vi "Frame create.vi"(7 "Command":string, 8 "error in (no error)":errorcluster, 11 "ISO 14443 B DOWN in":refnum<class "ISO 14443 B DOWN.lvclass">) -> (0 "error out":errorcluster, 3 "ISO 14443 B DOWN out":refnum<class "ISO 14443 B DOWN.lvclass">)   [LabVIEW 2019, in "ISO 14443 B DOWN.lvclass"]
uses:
  ISO 14443 B DOWN.lvclass
  TypeDef/Store.ctl
  ISO 14443 B DOWN.lvclass/ISO 14443 B DOWN.ctl
  RFID system.lvclass
panel:
  in  "APf":u8[](array[numeric])=[5] format="%x"
  in  "AFi":u8[](array[numeric])=[2] format="%x"
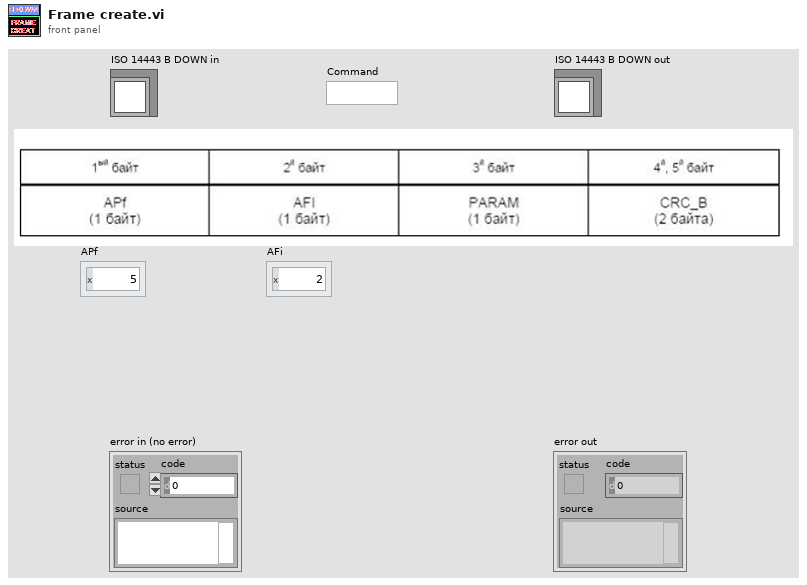
[diagram p1: front panel]
types:
  T1 = typedef "Store.ctl" = enum16{"envelope", "noise", "demSubCar", "CH_frame", "Decode", "demodulate", "in", "out", "sum", "subCarrier", "frame", "command", "encode", "modulate", "encode_UP", "modulate_up", "demod_up", "envelop_up", "sum_up", "out_up", "in_up"}
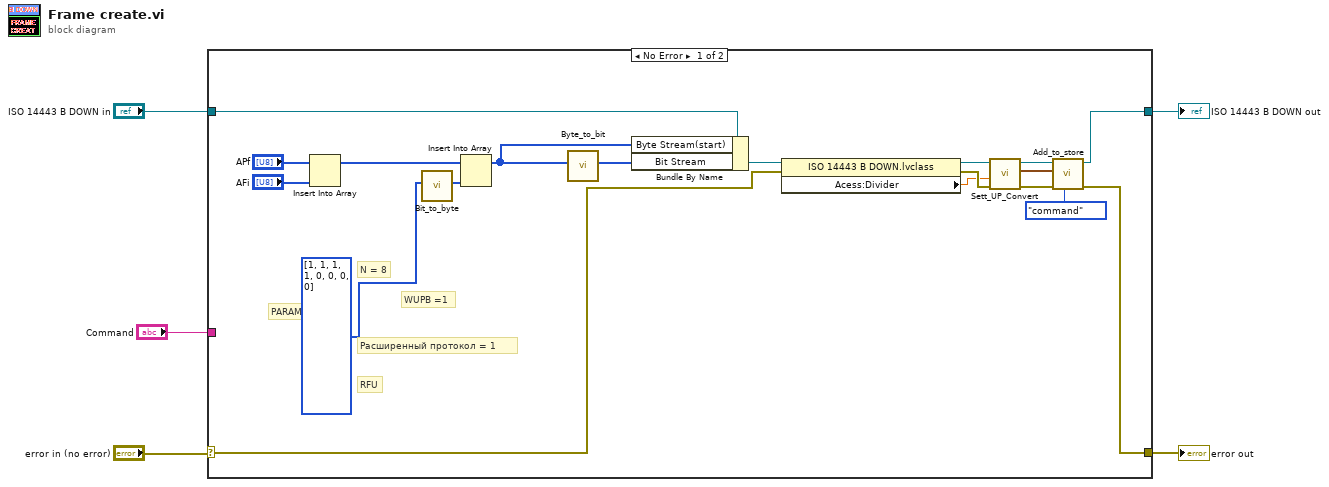
[diagram p0: block diagram]
diagram:
  n1 = case shown="No Error" "error in (no error)" {
    selector: "error in (no error)" -> [w12 w25]
    tunnel: "ISO 14443 B DOWN in" -> [w21 w26]
    tunnel: [w14 w26] -> w3
    tunnel: "Command" -> [_ _]
    tunnel: [w18 w25] -> w1
    frame No Error {
      # "PARAM"
      # "RFU"
      # "Расширенный протокол = 1"
      # "WUPB =1"
      # "N = 8"
      n2 = Insert Into Array(array="APf", new element="AFi") -> (w22:u8[])  [unwired: 1 in]
      n3 = call "Bit_to_byte.vi"("Array of bit"=u8[] [1, 1, 1, 1, 0, 0, 0, 0] ("AFi 2")) -> ("Array of byte"=w7:u8[])  [unwired: 8 in, 2 out]
      n4 = Insert Into Array(array=w22, new element=w7) -> (w6:u8[])  [unwired: 1 in]
      n5 = call "Byte_to_bit.vi"("Array of byte"=w6) -> ("Arrray of bit"=w8:u8[])  [unwired: 6 in, 2 out]
      n6 = Bundle By Name(cluster=w21, "Byte Stream(start)"=w6, "Bit Stream"=w8) -> (w20:refnum<class "ISO 14443 B DOWN.lvclass">)
      n7 = property class="ISO 14443 B DOWN.lvclass"(reference=w20, error in=w12) -> (reference out=w13:refnum<class "ISO 14443 B DOWN.lvclass">, error out=w11:errorcluster, "Acess:Divider"=w10:dbl)
      n8 = call-dynamic "Sett_UP_Convert.vi"("error in (no error)"=w11, "Divider(1)"=w10, "ISO 14443 B DOWN in"=w13) -> ("error out"=w19:errorcluster, "Waveform"=w15:waveform(dbl), "ISO 14443 B DOWN out"=w17:refnum<class "ISO 14443 B DOWN.lvclass">)  [unwired: 6 in]
      n9 = call "Add_to_store.vi"("Store"=Store."command", "error in (no error)"=w19, "Waveform"=w15, "RFID system in"=w17) -> ("error out"=w18:errorcluster, "RFID system out"=w14:refnum<class "ISO 14443 B DOWN.lvclass">)  [unwired: 6 in]
    }
    frame Error {
    }
  }
  "error out" <- w1
  "ISO 14443 B DOWN out" <- w3
